vi "CameraSetBinning.vi"(8 "error in (no error)":errorcluster, 9 "bin_y":u8, 10 "bin_x":u8, 11 "IMAQdx in":refnum<class "IMAQdx.lvclass">) -> (0 "error out":errorcluster, 2 "attribs":variant[](array[variant]), 3 "IMAQdx out":refnum<class "IMAQdx.lvclass">)   [LabVIEW 2010, in "IMAQdx.lvclass"]
uses:
  <userlib>/BIAS2/classes/IMAQdx/IMAQdx.lvclass
  <userlib>/BIAS2/classes/IMAQdx/IMAQdx.lvclass/IMAQdx.ctl
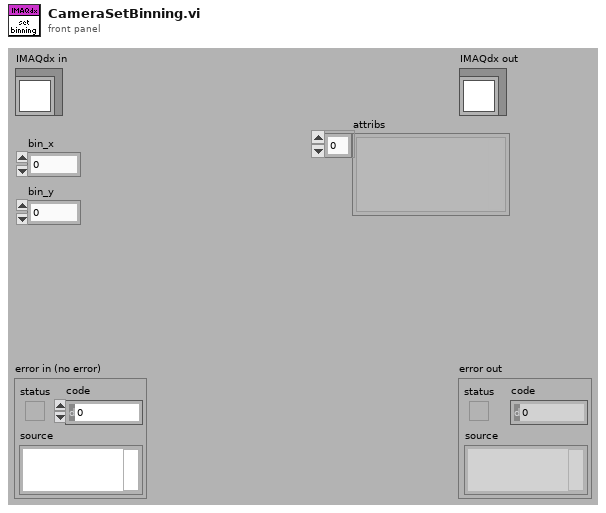
[diagram p1: front panel]
types:
  T1 = typedef "IMAQdx.ctl" = refnum<k21>
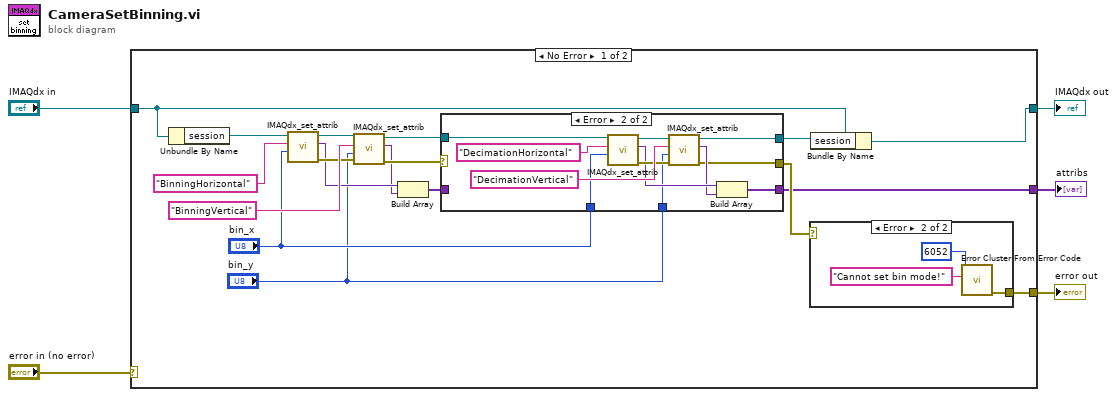
[diagram p0: block diagram]
diagram:
  n1 = case shown="No Error" "error in (no error)" {
    selector: "error in (no error)" -> [_ w43]
    tunnel: [w12 w43] -> w4
    tunnel: [w7 w42] -> w2
    tunnel: "IMAQdx in" -> [w8 w42]
    tunnel: [w11 _] -> w1
    frame No Error {
      n2 = Unbundle By Name(w8) -> ("session"=w23:refnum<k21>)
      n3 = call <userlib>:"IMAQdx_set_attrib.vi"("value"="bin_x", "attribute"="BinningHorizontal" ("ActiveAttribute"), "IMAQdx in"=w23) -> ("error out"=w18:errorcluster, "attrib out"=w16:variant, "IMAQdx out"=w22:T1)  [unwired: 2 in]
      n4 = call <userlib>:"IMAQdx_set_attrib.vi"("error in"=w18, "value"="bin_y", "attribute"="BinningVertical" ("ActiveAttribute"), "IMAQdx in"=w22) -> ("error out"=w17:errorcluster, "attrib out"=w15:variant, "IMAQdx out"=w21:T1)  [unwired: 1 in]
      n5 = Build Array(w16, w15) -> (w14:variant[])
      n6 = case shown="Error" w17 {
        selector: w17 -> [w28 _]
        tunnel: w21 -> [w27 w40]
        tunnel: w14 -> [w29 _]
        tunnel: [w29 w41] -> w11
        tunnel: [w28 w33] -> w13
        tunnel: "bin_x" -> [_ w32]
        tunnel: "bin_y" -> [_ w31]
        tunnel: [w27 w30] -> w6
        frame No Error {
        }
        frame Error {
          n7 = call <userlib>:"IMAQdx_set_attrib.vi"("value"=w32, "attribute"="DecimationHorizontal" ("ActiveAttribute"), "IMAQdx in"=w40) -> ("error out"=w36:errorcluster, "attrib out"=w35:variant, "IMAQdx out"=w38:T1)  [unwired: 2 in]
          n8 = call <userlib>:"IMAQdx_set_attrib.vi"("error in"=w36, "value"=w31, "attribute"="DecimationVertical" ("ActiveAttribute"), "IMAQdx in"=w38) -> ("error out"=w33:errorcluster, "attrib out"=w34:variant, "IMAQdx out"=w30:T1)  [unwired: 1 in]
          n9 = Build Array(w35, w34) -> (w41:variant[])
        }
      }
      n10 = case shown="Error" w13 {
        tunnel: [_ w26] -> w12
        frame No Error {
        }
        frame Error {
          n11 = call <vilib>:"Error Cluster From Error Code.vi"("error message (\"\")"="Cannot set bin mode!" ("error message (\"\")"), "error code (0)"=6052) -> ("error out"=w26:errorcluster)  [unwired: 7 in]
        }
      }
      n12 = Bundle By Name(cluster=w8, "session"=w6) -> (w7:refnum<class "IMAQdx.lvclass">)
    }
    frame Error {
    }
  }
  "error out" <- w4
  "IMAQdx out" <- w2
  "attribs" <- w1
